vi "Read Attribute.vi"(0 "Linked List in":refnum<class "Linked List.lvclass">, 1 "Linked List ID":string, 2 "Include Private?":bool, 3 "Flatten Pointer?":bool, 5 "Attribute Name":string, 9 "Type":variant, 11 "error in (no error)":errorcluster) -> (4 "Linked List out":refnum<class "Linked List.lvclass">, 6 "Attribute Name out":string, 10 "Attribute":variant, 12 "Found?":bool, 14 "Data ID":string, 15 "error out":errorcluster)   [LabVIEW 2017, in "Linked Lists.lvlib" / "Linked List.lvclass"]
uses:
  <vilib>/gpm_packages/@cs/linked-list/Source/Linked List/Linked List/Linked List.lvclass
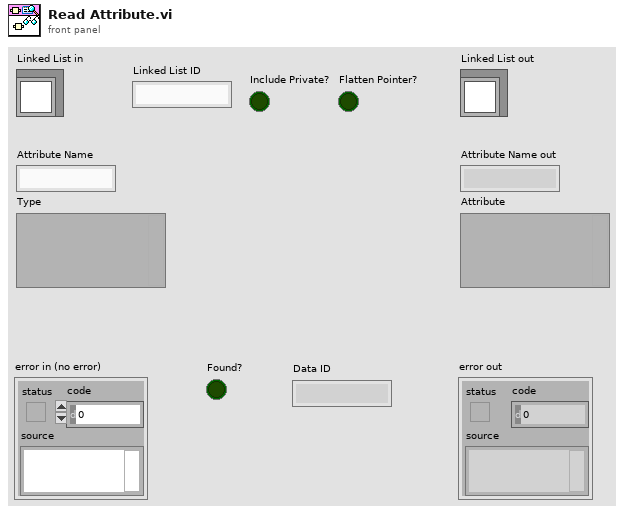
[diagram p1: front panel]
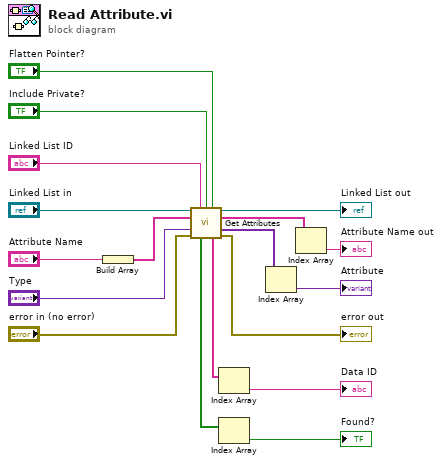
[diagram p0: block diagram]
diagram:
  n1 = Build Array("Attribute Name") -> (w14:string[])
  n2 = call <vilib>:"Get Attributes.vi"("Linked List in"="Linked List in", "Unique ID"="Linked List ID", "Include Private?"="Include Private?", "Flatten Pointer?"="Flatten Pointer?", "Attribute Names"=w14, "Type"="Type", "error in (no error)"="error in (no error)") -> ("Linked List out"=→"Linked List out":refnum<class "Linked List.lvclass">, "Attribute Names out"=w11:string[], "Attributes"=w9:variant[], "Found?"=w5:bool[], "Data IDs"=w7:string[], "error out"=→"error out":errorcluster)  [unwired: 2 in, 1 out]
  n3 = Index Array(array=w7) -> (element=→"Data ID":string)  [unwired: 1 in]
  n4 = Index Array(array=w5) -> (element=→"Found?":bool)  [unwired: 1 in]
  n5 = Index Array(array=w9) -> (element=→"Attribute":variant)  [unwired: 1 in]
  n6 = Index Array(array=w11) -> (element=→"Attribute Name out":string)  [unwired: 1 in]
